vi "流程大小.vi"(5 "功能":enum16{"写入", "读取"}(ring), 7 "大小":i32, 8 "error in (no error)":errorcluster caption="错误输入（无错误）", 11 "MB session in":refnum<class "MB_Master.lvclass">) -> (0 "error out":errorcluster caption="错误输出", 2 "大小读取":i32, 3 "MB session out":refnum<class "MB_Master.lvclass">)   [LabVIEW 2016, in "斯坦道总磷.lvlib"]
uses:
  <vilib>/Plasmionique/MB Master/MB_Master/MB_Master.lvclass
  <vilib>/Plasmionique/MB Master/MB Master.lvlib
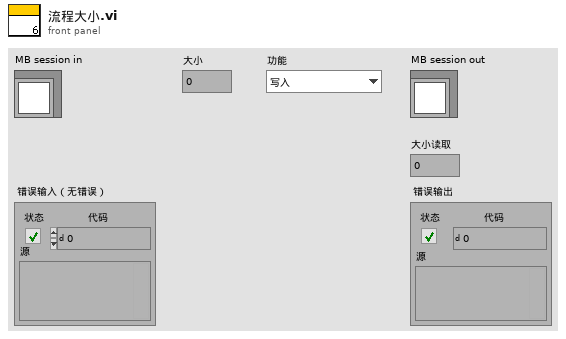
[diagram p1: front panel]
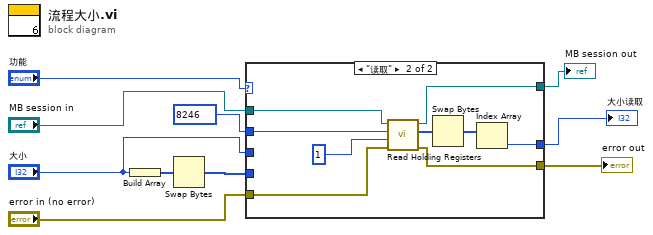
[diagram p0: block diagram]
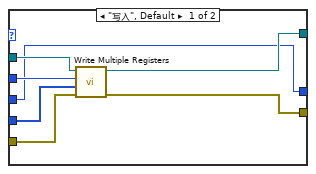
[diagram p2: hidden frame]
diagram:
  n1 = Build Array("大小") -> (w5:i32[])
  n2 = Swap Bytes(anything=w5) -> (byte swapped=w4:i32[])
  n3 = case shown="\"读取\"" "功能" {
    tunnel: "error in (no error)" -> [w17 w24]
    tunnel: [w16 w23] -> w9
    tunnel: [w15 w26] -> w8
    tunnel: u16 8246 ("starting address") -> [w14 w22]
    tunnel: "MB session in" -> [w13 w25]
    tunnel: w4 -> [w12 _]
    tunnel: [w11 w18] -> w1
    tunnel: "大小" -> [w11 _]
    frame "写入", Default {
      n4 = call <vilib>:"Write Multiple Registers.vi"("error in (no error)"=w17, "values"=w12, "starting address"=w14, "MB session in"=w13) -> ("error out"=w16:errorcluster, "MB session out"=w15:refnum<class "MB_Master.lvclass">)  [unwired: 6 in]
    }
    frame "读取" {
      n5 = call <vilib>:"Read Holding Registers.vi"("error in (no error)"=w24, "quantity"=u16 1, "starting address"=w22, "MB session in"=w25) -> ("error out"=w23:errorcluster, "Registers"=w20:u16[], "MB session out"=w26:refnum<class "MB_Master.lvclass">)  [unwired: 5 in]
      n6 = Swap Bytes(anything=w20) -> (byte swapped=w19:u16[])
      n7 = Index Array(array=w19) -> (element=w18:u16)  [unwired: 1 in]
    }
  }
  "error out" <- w9
  "MB session out" <- w8
  "大小读取" <- w1
